vi "UPS_CalculateDowntime.vi"(4 "Init?":bool, 5 "Prsnt?":bool) -> (1 "Downtime(s)":dbl)   [LabVIEW 2018]
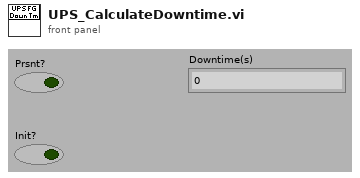
[diagram p1: front panel]
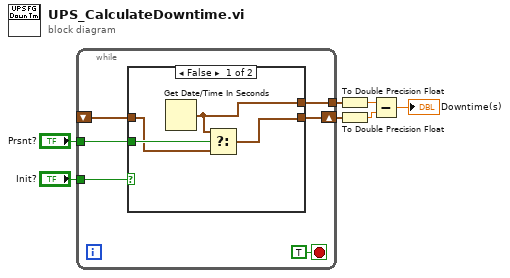
[diagram p0: block diagram]
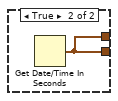
[diagram p2: hidden frame]
diagram:
  n1 = while {
    shift-right: [w11] -> w4
    shift-left: _ -> [w10]
    tunnel: "Prsnt?" -> [w12]
    tunnel: "Init?" -> [w9]
    tunnel: [w8] -> w5
    stop <- TRUE ("Boolean") stop-if-true
    n2 = case shown="False" w9 {
      tunnel: w12 -> [w17 _]
      tunnel: [w16 w18] -> w11
      tunnel: w10 -> [w15 _]
      tunnel: [w14 w18] -> w8
      frame False {
        n3 = Get Date/Time In Seconds() -> (seconds since 1Jan1904=w14:timestamp)
        n4 = Select(t=w14, s=w17, f=w15) -> (s? t:f=w16:timestamp)
      }
      frame True {
        n5 = Get Date/Time In Seconds() -> (seconds since 1Jan1904=w18:timestamp)
      }
    }
  }
  n6 = To Double Precision Float(number=w5) -> (double precision float=w3:dbl)
  n7 = To Double Precision Float(number=w4) -> (double precision float=w2:dbl)
  n8 = Subtract(x=w3, y=w2) -> (x-y=→"Downtime(s)":dbl)
